vi "test_check.vi"() -> ()   [LabVIEW 2017]
panel:
  out "data":bool
  in  "use":bool
  in  "add":bool
  in  "ini":bool
  in  "stop":bool
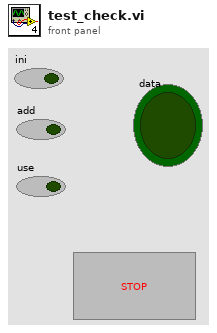
[diagram p1: front panel]
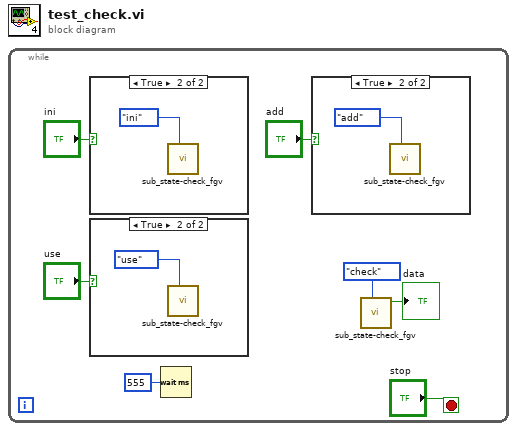
[diagram p0: block diagram]
diagram:
  n1 = while {
    stop <- "stop" stop-if-true
    n2 = case shown="True" "ini" {
      frame False {
      }
      frame True {
        n3 = call "sub_state-check_fgv.vi"("cmd"=enum16{"ini", "add", "use", "check"}."ini") -> ()  [unwired: 9 in, 2 out]
      }
    }
    n4 = case shown="True" "use" {
      frame False {
      }
      frame True {
        n5 = call "sub_state-check_fgv.vi"("cmd"=enum16{"ini", "add", "use", "check"}."use") -> ()  [unwired: 9 in, 2 out]
      }
    }
    n6 = Wait (ms)(milliseconds to wait=u32 555) -> ()  [unwired: 1 out]
    n7 = case shown="True" "add" {
      frame False {
      }
      frame True {
        n8 = call "sub_state-check_fgv.vi"("cmd"=enum16{"ini", "add", "use", "check"}."add") -> ()  [unwired: 9 in, 2 out]
      }
    }
    n9 = call "sub_state-check_fgv.vi"("cmd"=enum16{"ini", "add", "use", "check"}."check") -> ("data"=→"data":bool)  [unwired: 9 in, 1 out]
  }
